vi "Identify.vi"(8 "error in (no error)":errorcluster, 11 "Triangle in":refnum<class "Triangle.lvclass">) -> (0 "error out":errorcluster, 2 "Class name":string, 3 "Triangle out":refnum<class "Triangle.lvclass">)   [LabVIEW 2023, in "Triangle.lvclass"]
doc: "This VI is a method that demonstrates dynamic dispatching."
uses:
  Triangle.lvclass
panel:
  in  "Class name (constant)":string="Triangle"
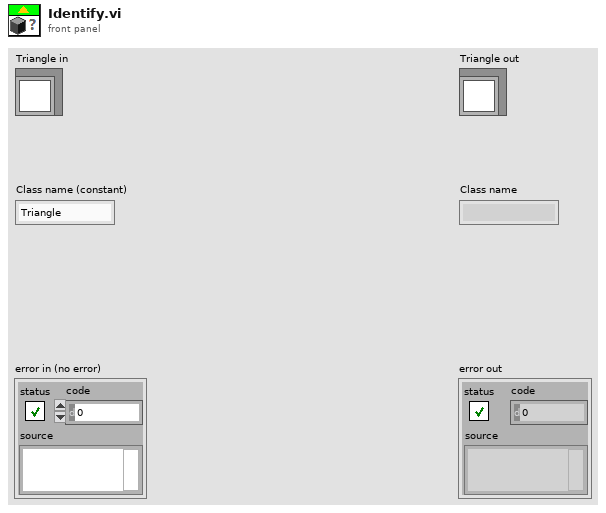
[diagram p1: front panel]
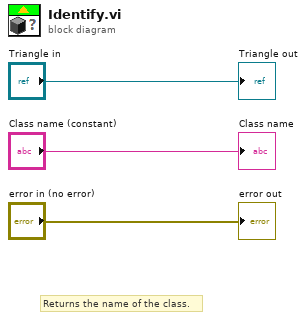
[diagram p0: block diagram]
diagram:
  # "Returns the name of the class."
  "error out" <- "error in (no error)"
  "Triangle out" <- "Triangle in"
  "Class name" <- "Class name (constant)"
